vi "handleIRQ.vi"(8 "error in (no error)":errorcluster, 10 "fpgaVIRefCRIO9074":T1, 11 "IRQHandler in":refnum<class "IRQHandler.lvclass">) -> (0 "error out":errorcluster, 3 "IRQHandler out":refnum<class "IRQHandler.lvclass">)   [LabVIEW 2013, in "ComponentData.lvlib" / "IRQHandler.lvclass"]
uses:
  <userlib>/Common/Component/common_application/RT/ComponentData/IRQHandler/IRQHandler.lvclass
  <userlib>/Common/Component/common_application/RT/ComponentData/ComponentData/fpgaVIRefCRIO9074.ctl
  <userlib>/Common/Component/common_application/RT/ComponentData/IRQHandler/IRQHandler.lvclass/IRQHandler.ctl
  <vilib>/rvi/interface/common/niFpgaWaitOnOcc.vi
  <vilib>/Utility/error.llb/Error Cluster From Error Code.vi
  <vilib>/RVI Host/nirviSupport.llb/nirviErrorClusterFromErrorCode.vi
  <vilib>/rvi/errors/niLvFpgaAdjustHostInterfaceError.vi
  <vilib>/rvi/interface/nirviMethod/nirviMethod.xnode
  <userlib>/Common/Component/common_application/RT/ComponentData/ConfigurationHandler/IRQConfig/IRQConfig.lvclass
  <userlib>/Common/Component/common_application/RT/ComponentData.lvlib
  <vilib>/rvi/interface/nirviMethod/StockFPGA_InlinedMethodWaitForSingleIRQ.vi
  <vilib>/FPGAPlugInAG/cRIO-9074/niLvFpga_WaitOnIrq_cRIO-9074.vi
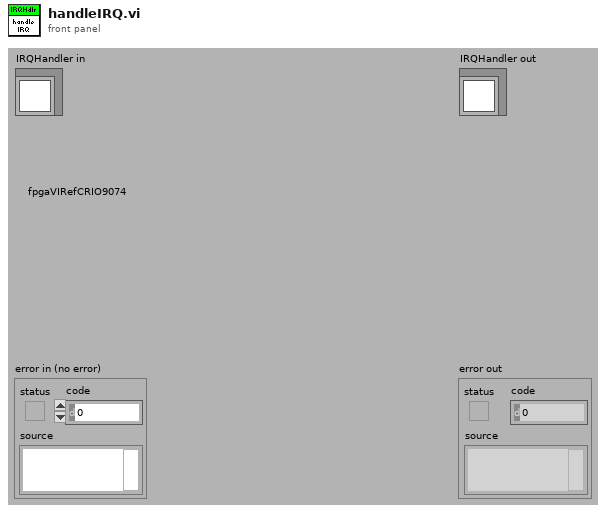
[diagram p1: front panel]
types:
  T1 = typedef "ComponentData.lvlib/fpgaVIRefCRIO9074.ctl" = refnum<k20>
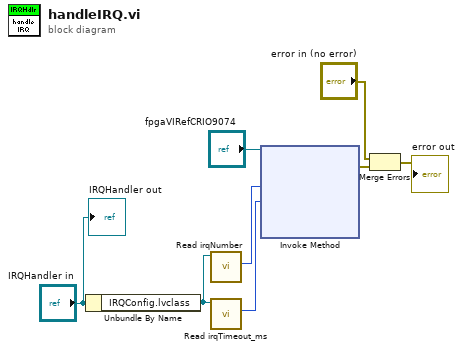
[diagram p0: block diagram]
diagram:
  n1 = Unbundle By Name("IRQHandler in") -> ("IRQConfig.lvclass"=w7:refnum<class "IRQConfig.lvclass">)
  n2 = call <userlib>:"Read irqNumber.vi"("IRQConfig in"=w7) -> ("irqNumber"=w5:i32)  [unwired: 8 in, 2 out]
  n3 = call <userlib>:"Read irqTimeout_ms.vi"("IRQConfig in"=w7) -> ("irqTimeout_ms"=w4:i32)  [unwired: 8 in, 2 out]
  n4 = xnode "Invoke Method"("FPGA VI Reference In"="fpgaVIRefCRIO9074", "IRQ Number(s)"=w5, "Timeout (ms)"=w4) -> ("error out"=w2:errorcluster)  [unwired: 1 in, 3 out]
  n5 = Merge Errors("error in (no error)", w2) -> (→"error out":errorcluster)
  "IRQHandler out" <- "IRQHandler in"
